vi "Pather.vi"(7 "Array 2":refnum<vi>, 10 "output array":T1[][](array[typedef])) -> ()   [LabVIEW 2016]
uses:
  Controls/TileColor.ctl
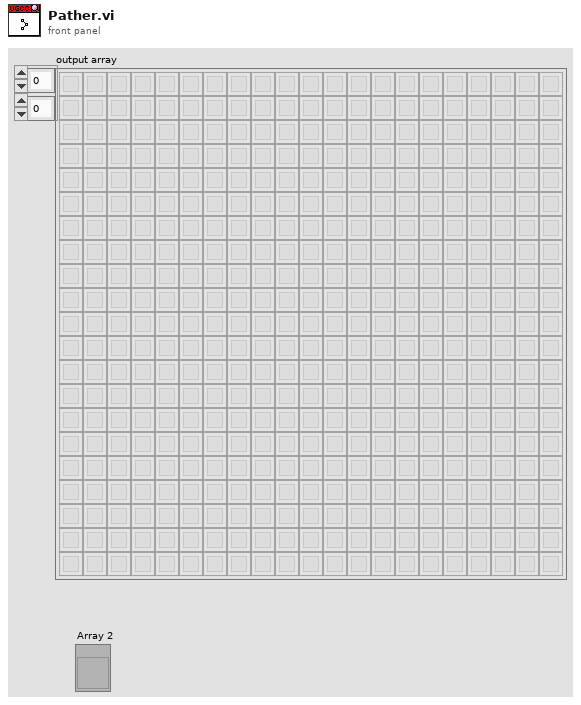
[diagram p1: front panel]
types:
  T1 = typedef "TileColor.ctl" = u16
  T2 = typedef "Parse-(X,Y).ctl" = cluster{"X":i32, "Y":i32, "Tile Color":T1}
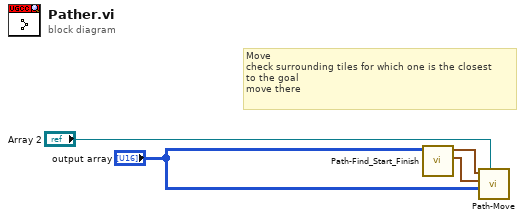
[diagram p0: block diagram]
diagram:
  # "Move\ncheck surrounding tiles for which one is the closest\nto the goal\nmove there"
  n1 = call "Path-Find_Start_Finish.vi"("Tile Array"="output array") -> ("Start"=w3:T2, "Finish"=w4:T2)  [unwired: 9 in]
  n2 = call "Path-Move.vi"("Maze Display Ref"="Array 2", "Tile Array"="output array", "Start"=w3, "Finish"=w4) -> ()  [unwired: 7 in, 1 out]
